vi "BoP Output Client.vi"() -> ()   [LabVIEW 2017]
uses:
  <vilib>/OPCUA/controls/Write Status.ctl
  <vilib>/OPCUA/controls/NodeId.ctl
  <vilib>/OPCUA/client/Multiple Write Double Array.vi
  <vilib>/OPCUA/NI OPC UA Client.lvlib
panel:
  in  "Stop BoP Output Writing":bool
  in  "Time Stamp":timestamp
  in  "Node Status":T1 items=["Good"=0, "Uncertain_InitialValue"=1083310080, "Uncertain_LastUsableValue"=1083179008, "Uncertain_SensorNotAccurate"=1083375616, "Uncertain_EngineeringUnitsExceeded"=1083441152, "Bad_NoCommunication"=2150694912, "Bad_NotReadable"=2151284736, "Bad_NotWritable"=2151350272, "Bad_OutOfRange"=2151415808, "Bad_WaitingForInitialData"=2150760448]
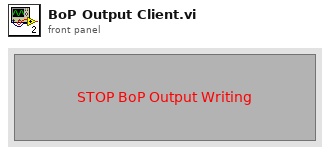
[diagram p1: front panel]
types:
  T1 = typedef "Write Status.ctl" = u32
  T2 = cluster{"message mode":enum16{"None", "Sign", "Sign and Encrypt"}, "security":enum16{"Basic256", "Basic128Rsa15"}}
  T3 = typedef "OPC UA Client Refnum.ctl" = refnum<k21>
  T4 = typedef "NodeId.ctl" = string
  T5 = cluster{"node ID":T4, "value":dbl[], "timestamp (current time)":timestamp, "node status":T1}
  T6 = cluster{"node ID":T4, "value":dbl[], "timestamp (current time)":timestamp, "node status":T1}[]
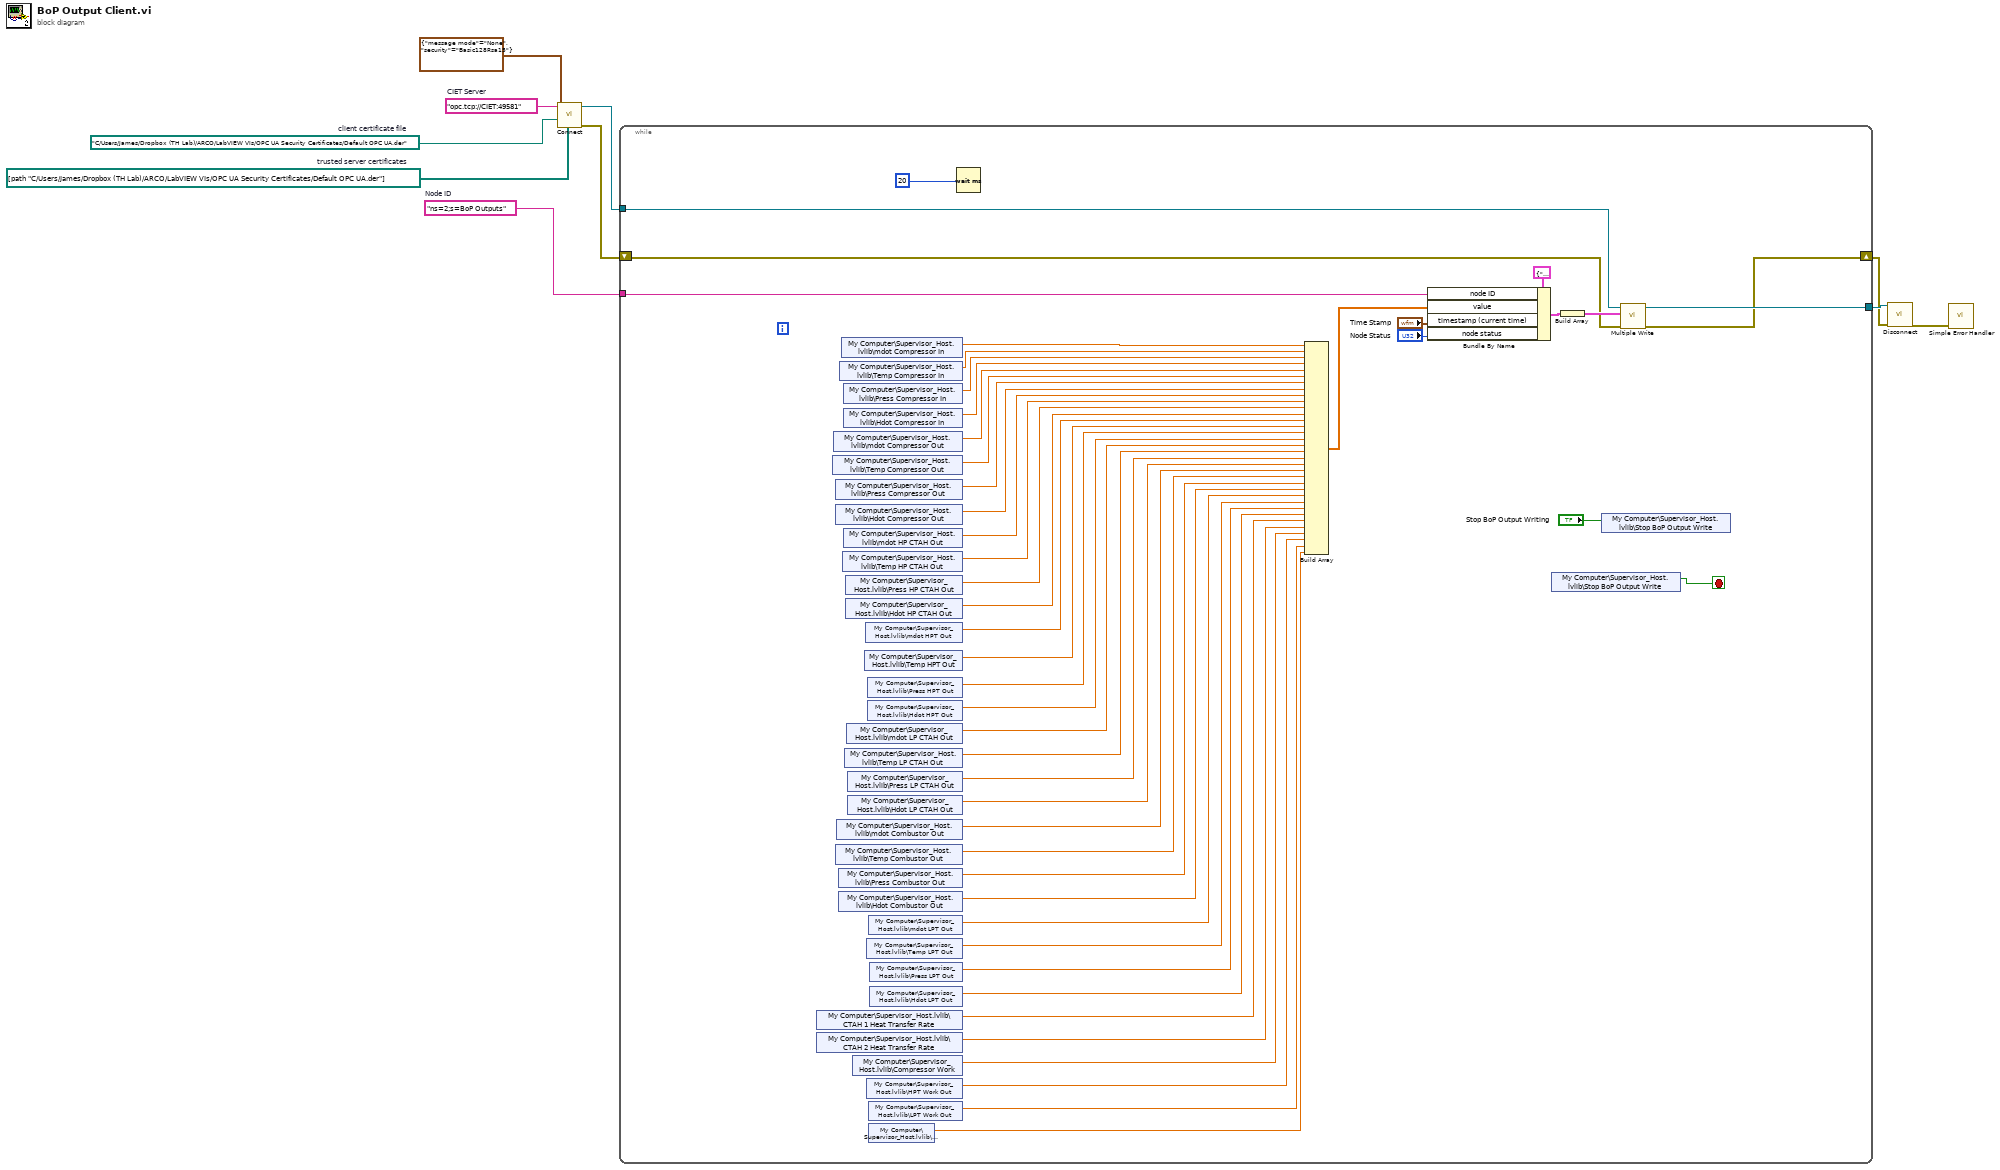
[diagram p0: block diagram]
diagram:
  w4 = path[] [path "C:/Users/James/Dropbox (TH Lab)/ARCO/LabVIEW VIs/OPC UA Security Certificates/Default OPC UA.der"]  # trusted server certificates
  w5 = path "C:/Users/James/Dropbox (TH Lab)/ARCO/LabVIEW VIs/OPC UA Security Certificates/Default OPC UA.der"  # client certificate file
  w7 = "ns=2;s=BoP Outputs"  # Node ID
  w9 = "opc.tcp://CIET:49581"  # CIET Server
  n1 = call <vilib>:"Connect.vi"("trusted server certificates"=w4, "client certificate file"=w5, "security policy"=T2 {"message mode"=enum."None", "security"=enum."Basic128Rsa15"}, "server endpoint URL"=w9) -> ("error out"=w2:errorcluster, "OPC UA client refnum out"=w8:T3)  [unwired: 5 in, 1 out]
  n2 = while {
    tunnel: w7 -> [w57]
    tunnel: w8 -> [w55]
    tunnel: [w56] -> w6
    shift-right: [w49] -> w1
    shift-left: w2 -> [w48]
    stop <- w18 stop-if-true
    n3 = shared-variable "My Computer\\Supervisor_Host.lvlib\\CTAH 1 Heat Transfer Rate"() -> (w16:sgl)  [unwired: 1 in, 1 out]
    n4 = shared-variable "My Computer\\Supervisor_Host.lvlib\\CTAH 2 Heat Transfer Rate"() -> (w15:sgl)  [unwired: 1 in, 1 out]
    n5 = shared-variable "My Computer\\Supervisor_Host.lvlib\\Temp Compressor Out"() -> (w40:sgl)  [unwired: 1 in, 1 out]
    n6 = shared-variable "My Computer\\Supervisor_Host.lvlib\\mdot Compressor Out"() -> (w42:sgl)  [unwired: 1 in, 1 out]
    n7 = shared-variable "My Computer\\Supervisor_Host.lvlib\\Press Compressor Out"() -> (w41:sgl)  [unwired: 1 in, 1 out]
    n8 = shared-variable "My Computer\\Supervisor_Host.lvlib\\Hdot Compressor Out"() -> (w39:sgl)  [unwired: 1 in, 1 out]
    n9 = shared-variable "My Computer\\Supervisor_Host.lvlib\\Temp Combustor Out"() -> (w26:sgl)  [unwired: 1 in, 1 out]
    n10 = shared-variable "My Computer\\Supervisor_Host.lvlib\\mdot Combustor Out"() -> (w27:sgl)  [unwired: 1 in, 1 out]
    n11 = shared-variable "My Computer\\Supervisor_Host.lvlib\\Press Combustor Out"() -> (w25:sgl)  [unwired: 1 in, 1 out]
    n12 = shared-variable "My Computer\\Supervisor_Host.lvlib\\Hdot Combustor Out"() -> (w24:sgl)  [unwired: 1 in, 1 out]
    n13 = shared-variable "My Computer\\Supervisor_Host.lvlib\\Temp Compressor In"() -> (w45:sgl)  [unwired: 1 in, 1 out]
    n14 = shared-variable "My Computer\\Supervisor_Host.lvlib\\mdot Compressor In"() -> (w46:sgl)  [unwired: 1 in, 1 out]
    n15 = shared-variable "My Computer\\Supervisor_Host.lvlib\\Temp HP CTAH Out"() -> (w37:sgl)  [unwired: 1 in, 1 out]
    n16 = shared-variable "My Computer\\Supervisor_Host.lvlib\\Press Compressor In"() -> (w44:sgl)  [unwired: 1 in, 1 out]
    n17 = shared-variable "My Computer\\Supervisor_Host.lvlib\\Hdot Compressor In"() -> (w43:sgl)  [unwired: 1 in, 1 out]
    n18 = shared-variable "My Computer\\Supervisor_Host.lvlib\\mdot HP CTAH Out"() -> (w38:sgl)  [unwired: 1 in, 1 out]
    n19 = shared-variable "My Computer\\Supervisor_Host.lvlib\\Temp LP CTAH Out"() -> (w30:sgl)  [unwired: 1 in, 1 out]
    n20 = shared-variable "My Computer\\Supervisor_Host.lvlib\\Press HP CTAH Out"() -> (w36:sgl)  [unwired: 1 in, 1 out]
    n21 = shared-variable "My Computer\\Supervisor_Host.lvlib\\Hdot HP CTAH Out"() -> (w35:sgl)  [unwired: 1 in, 1 out]
    n22 = shared-variable "My Computer\\Supervisor_Host.lvlib\\mdot LP CTAH Out"() -> (w31:sgl)  [unwired: 1 in, 1 out]
    n23 = shared-variable "My Computer\\Supervisor_Host.lvlib\\Press LP CTAH Out"() -> (w29:sgl)  [unwired: 1 in, 1 out]
    n24 = shared-variable "My Computer\\Supervisor_Host.lvlib\\Hdot LP CTAH Out"() -> (w28:sgl)  [unwired: 1 in, 1 out]
    n25 = shared-variable "My Computer\\Supervisor_Host.lvlib\\Compressor Work"() -> (w14:sgl)  [unwired: 1 in, 1 out]
    n26 = shared-variable "My Computer\\Supervisor_Host.lvlib\\Temp HPT Out"() -> (w34:sgl)  [unwired: 1 in, 1 out]
    n27 = shared-variable "My Computer\\Supervisor_Host.lvlib\\mdot HPT Out"() -> (w19:sgl)  [unwired: 1 in, 1 out]
    n28 = shared-variable "My Computer\\Supervisor_Host.lvlib\\Temp LPT Out"() -> (w22:sgl)  [unwired: 1 in, 1 out]
    n29 = shared-variable "My Computer\\Supervisor_Host.lvlib\\HPT Work Out"() -> (w13:sgl)  [unwired: 1 in, 1 out]
    n30 = shared-variable "My Computer\\Supervisor_Host.lvlib\\Press HPT Out"() -> (w33:sgl)  [unwired: 1 in, 1 out]
    n31 = shared-variable "My Computer\\Supervisor_Host.lvlib\\Hdot HPT Out"() -> (w32:sgl)  [unwired: 1 in, 1 out]
    n32 = shared-variable "My Computer\\Supervisor_Host.lvlib\\mdot LPT Out"() -> (w23:sgl)  [unwired: 1 in, 1 out]
    n33 = shared-variable "My Computer\\Supervisor_Host.lvlib\\LPT Work Out"() -> (w12:sgl)  [unwired: 1 in, 1 out]
    n34 = shared-variable "My Computer\\Supervisor_Host.lvlib\\Time_R"() -> (w11:sgl)  [unwired: 1 in, 1 out]
    n35 = shared-variable "My Computer\\Supervisor_Host.lvlib\\Press LPT Out"() -> (w21:sgl)  [unwired: 1 in, 1 out]
    n36 = shared-variable "My Computer\\Supervisor_Host.lvlib\\Hdot LPT Out"() -> (w20:sgl)  [unwired: 1 in, 1 out]
    n37 = Wait (ms)(milliseconds to wait=u32 20) -> ()  [unwired: 1 out]
    n38 = Build Array(w46, w45, w44, w43, w42, w40, w41, w39, w38, w37, w36, w35, w19, w34, w33, w32, w31, w30, w29, w28, w27, w26, w25, w24, w23, w22, w21, w20, w16, w15, w14, w13, w12, w11) -> (w47:sgl[])
    n39 = Bundle By Name(cluster=T5 {"node ID"="", "value"=[], "timestamp (current time)"=timestamp(0 s since 1904-01-01), "node status"=0} ("request"), "node ID"=w57, "value"=w47, "timestamp (current time)"="Time Stamp", "node status"="Node Status") -> (w51:T5)
    n40 = shared-variable "My Computer\\Supervisor_Host.lvlib\\Stop BoP Output Write"() -> (w18:bool)  [unwired: 1 in, 1 out]
    n41 = Build Array(w51) -> (w50:T6)
    n42 = shared-variable "My Computer\\Supervisor_Host.lvlib\\Stop BoP Output Write"("Stop BoP Output Writing") -> ()  [unwired: 1 in, 1 out]
    n43 = call-poly <vilib>:"Multiple Write.vi"("error in (no error)"=w48, "requests"=w50, "OPC UA client refnum in"=w55) -> ("error out"=w49:errorcluster, "OPC UA client refnum out"=w56:T3)  [unwired: 5 in, 2 out]
  }
  n44 = call <vilib>:"Disconnect.vi"("error in (no error)"=w1, "OPC UA client refnum in"=w6) -> ("error out"=w10:errorcluster)  [unwired: 9 in]
  n45 = call <vilib>:"Simple Error Handler.vi"("error in (no error)"=w10) -> ()  [unwired: 4 in, 5 out]
